vi "Get Translation.vi"(8 "error in (no error)":errorcluster, 11 "Scene Object":refnum<vi>) -> (0 "error out":errorcluster, 2 "Transformation:Get Translation":cluster{"X":sgl, "Y":sgl, "Z":sgl}, 3 "Scene Object":refnum<vi>)   [LabVIEW 2020, in "NI_3D Picture Control.lvlib"]
doc: "Returns the translation applied to an object in a 3D scene."
uses:
  <vilib>/picture/3D Picture Control/NI_3D Picture Control.lvlib
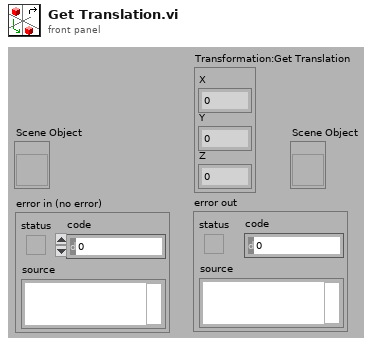
[diagram p1: front panel]
types:
  T1 = typedef "LV3DPointTypeDef.ctl" = cluster{"X":sgl, "Y":sgl, "Z":sgl}
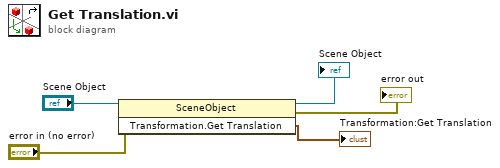
[diagram p0: block diagram]
diagram:
  n1 = invoke class="SceneObject" method="Transformation.Get Translation"(reference="Scene Object", error in="error in (no error)") -> (reference out=→"Scene Object":refnum<vi>, error out=→"error out":errorcluster, "Transformation.GetTranslation"=→"Transformation:Get Translation":T1)  [unwired: 1 in]
